vi "Create File.vi"(8 "error in (no error)":errorcluster, 10 "File Name Prefix":string) -> (0 "error out":errorcluster, 3 "refnum out":refnum<file>)   [LabVIEW 2015]
uses:
  <vilib>/Utility/sysdir.llb/System Directory Type.ctl
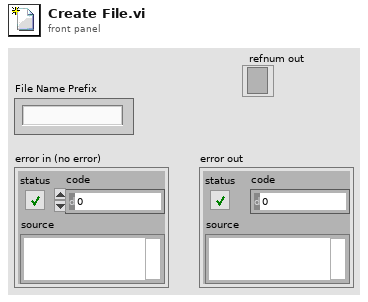
[diagram p1: front panel]
types:
  T1 = typedef "System Directory Type.ctl" = i32
  T2 = enum16{"open", "replace", "create", "open or create", "replace or create", "replace or create with confirmation"}
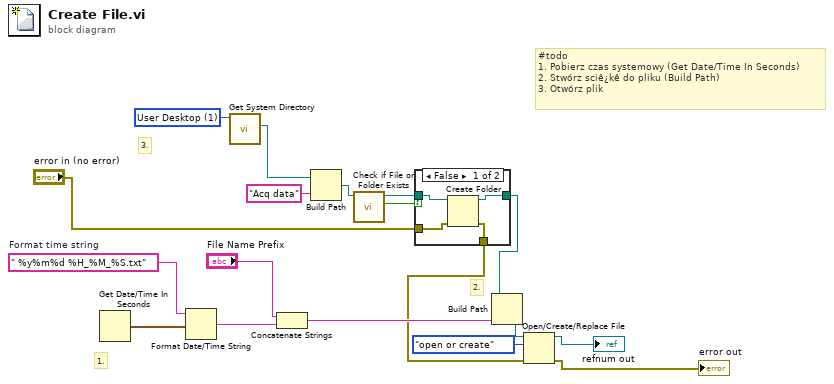
[diagram p0: block diagram]
diagram:
  w10 = T1 1 items=["User Home"=0, "User Desktop"=1, "User Documents"=2, "User Application Data"=3, "User Preferences"=4, "User Temporary"=5, "Public Documents"=6, "Public Application Data"=7, "Public Preferences"=8, "Public Cache"=13, "System Core Libraries"=9, "System Installed Libraries"=10, "Application Files"=11, "Boot Volume Root"=12] ("system directory type")
  w17 = " %y%m%d %H_%M_%S.txt"  # Format time string
  # "3."
  # "2."
  # "1."
  # "#todo\n1. Pobierz czas systemowy (Get Date/Time In Seconds)\n2. Stwórz sciê¿kê do pliku (Build Path)\n3. Otwórz plik"
  n1 = Get Date/Time In Seconds() -> (seconds since 1Jan1904=w15:timestamp)
  n2 = Format Date/Time String(time format string (%c)=w17, seconds (now)=w15) -> (date/time string=w18:string)  [unwired: 1 in]
  n3 = call <vilib>:"Get System Directory.vi"("system directory type"=w10) -> ("system directory"=w8:path)  [unwired: 10 in]
  n4 = Concatenate Strings("File Name Prefix", w18) -> (w13:string)
  n5 = Build Path(base path=w8, name or relative path="Acq data") -> (appended path=w4:path)
  n6 = call <vilib>:"Check if File or Folder Exists.vi"("path"=w4) -> ("file or folder exists?"=w6:bool, "dup path"=w5:path)  [unwired: 8 in, 1 out]
  n7 = case shown="False" w6 {
    tunnel: w5 -> [w22 w24]
    tunnel: [w21 w24] -> w3
    tunnel: "error in (no error)" -> [w20 w23]
    tunnel: [w19 w23] -> w1
    frame False {
      n8 = Create Folder(path (use dialog)=w22, error in=w20) -> (created path=w21:path, error out=w19:errorcluster)  [unwired: 1 in, 1 out]
    }
    frame True {
    }
  }
  n9 = Build Path(base path=w3, name or relative path=w13) -> (appended path=w9:path)
  n10 = Open/Create/Replace File(file path (use dialog)=w9, error in=w1, operation (0:open)=T2."open or create") -> (refnum out=→"refnum out":refnum<file>, error out=→"error out":errorcluster)  [unwired: 3 in, 1 out]
